vi "温度计变色显示.vi"() -> ()   [LabVIEW 2012]
panel:
  out "温度计":dbl(slide) scale=20.0..30.0
  # "说明：\n温度＞28℃  红色\n温度＞23℃  蓝色\n温度在23℃与28℃之间  绿色"
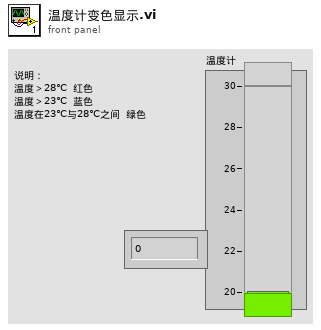
[diagram p1: front panel]
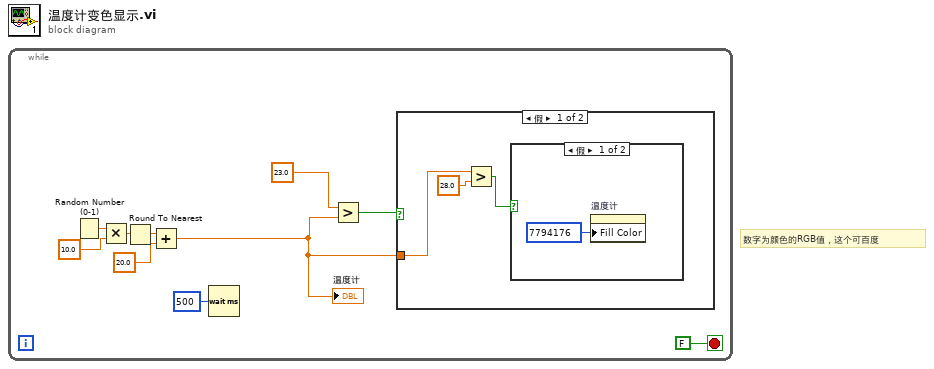
[diagram p0: block diagram]
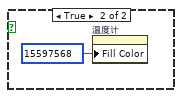
[diagram p2: hidden frame]
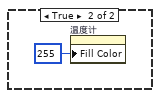
[diagram p3: hidden frame]
diagram:
  # "数字为颜色的RGB值，这个可百度"
  n1 = while {
    stop <- FALSE stop-if-true
    n2 = Random Number (0-1)() -> (number: 0 to 1=w8:dbl)
    n3 = Multiply(x=w8, y=10.0) -> (x*y=w9:dbl)
    n4 = Round To Nearest(number=w9) -> (nearest integer value=w6:dbl)
    n5 = Add(x=w6, y=20.0) -> (x+y=w1:dbl)
    "温度计" <- w1
    n6 = Wait (ms)(milliseconds to wait=u32 500 ("等待时间（毫秒）")) -> ()  [unwired: 1 out]
    n7 = Greater?(x=23.0, y=w1) -> (0:w2:bool)
    n8 = case shown="假" w2 {
      tunnel: w1 -> [w13 _]
      frame False {
        n9 = Greater?(x=w13, y=28.0) -> (0:w11:bool)
        n10 = case shown="假" w11 {
          frame False {
            n11 = property on="温度计" class="Slide (严格)"("Fill Color"=u32 7794176 ("填充颜色")) -> ()  [unwired: 2 in, 2 out]
          }
          frame True {
            n12 = property on="温度计" class="Slide (严格)"("Fill Color"=u32 15597568 ("填充颜色")) -> ()  [unwired: 2 in, 2 out]
          }
        }
      }
      frame True {
        n13 = property on="温度计" class="Slide (严格)"("Fill Color"=u32 255 ("填充颜色")) -> ()  [unwired: 2 in, 2 out]
      }
    }
  }
